vi "Elevation.vi"(0 "SP (degrees)":dbl=60.0, 5 "P-gain":dbl=1e-05, 7 "Deadband (degrees)":dbl=5.0, 11 "error in (no error)":errorcluster) -> (3 "Elevation Motor":dbl, 4 "PV (degrees)":dbl, 14 "Elevation OK?":bool, 15 "error out":errorcluster)   [LabVIEW 2016]
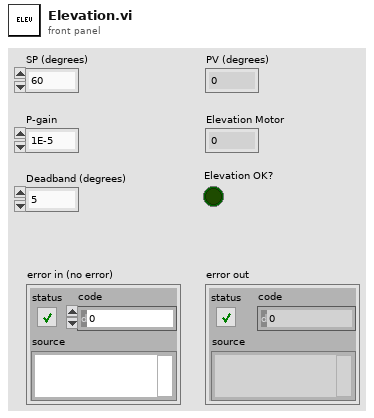
[diagram p1: front panel]
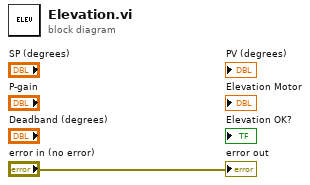
[diagram p0: block diagram]
diagram:
  "error out" <- "error in (no error)"
